vi "tower Check for New Command.vi"(8 "Current Command":T6, 10 "Wait time (ms)":dbl, 11 "Finished?":bool) -> (0 "Completion":T4, 1 "Subsystem Name":string, 2 "Current Command":T1, 3 "Initial Trace String":string, 4 "NextCommand":T6)   [LabVIEW 2017]
doc: "This VI is called for each controller loop iteration. It checks for new commands, updates timing data, and upon completion, notifies any waiting commands."
uses:
  tower Setpoints.ctl
  tower Operations.ctl
  <vilib>/Rock Robotics/WPI/Framework/Command Status Info.ctl
  <vilib>/Rock Robotics/WPI/Framework/Completion Status.ctl
  <vilib>/Rock Robotics/WPI/Framework/Completion Notifier.ctl
  tower Published Globals.vi
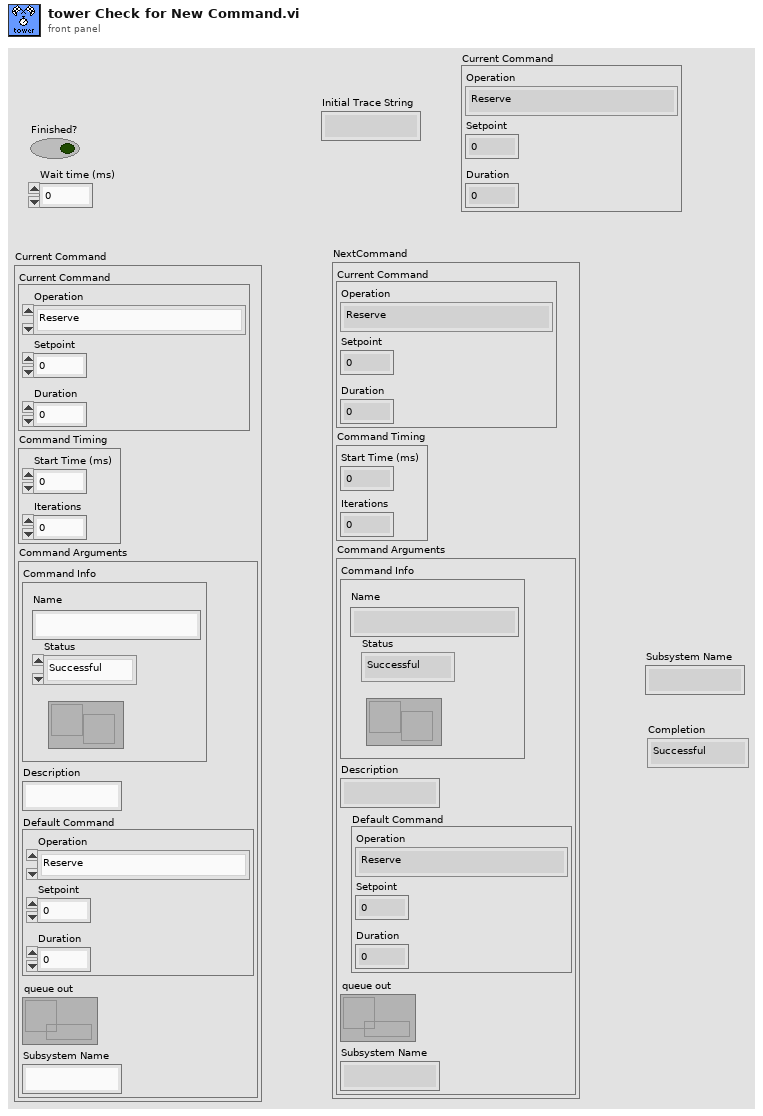
[diagram p1: front panel]
types:
  T1 = typedef "tower Setpoints.ctl" = cluster{"Operation":T2, "Setpoint":dbl, "Duration":dbl}
  T2 = typedef "tower Operations.ctl" = enum16{"Reserve", "Read Current", "Immediate", "LaunchClimber", "ArmReset", "ArmPosition", "TowerClimbImmediate", "ArmSpitPosition", "ClimbArmMove"}
  T3 = typedef "Command Status Info.ctl" = cluster{"Name":string, "Status":T4, "notifier out":T5}
  T4 = typedef "Completion Status.ctl" = enum16{"Successful", "Aborted", "Incomplete"}
  T5 = typedef "Completion Notifier.ctl" = refnum<notifier>
  T6 = cluster{"Current Command":T1, "Command Timing":cluster{"Start Time (ms)":u32, "Iterations":i32}, "Command Arguments":cluster{"Command Info":T3, "Description":string, "Default Command":T1, "queue out":refnum<queue>, "Subsystem Name":string}}
  T7 = cluster{"Command Info":T3, "Description":string, "Default Command":T1, "queue out":refnum<queue>, "Subsystem Name":string}
  T8 = cluster{"Default Command":T1, "Command Info":T3, "Description":string}
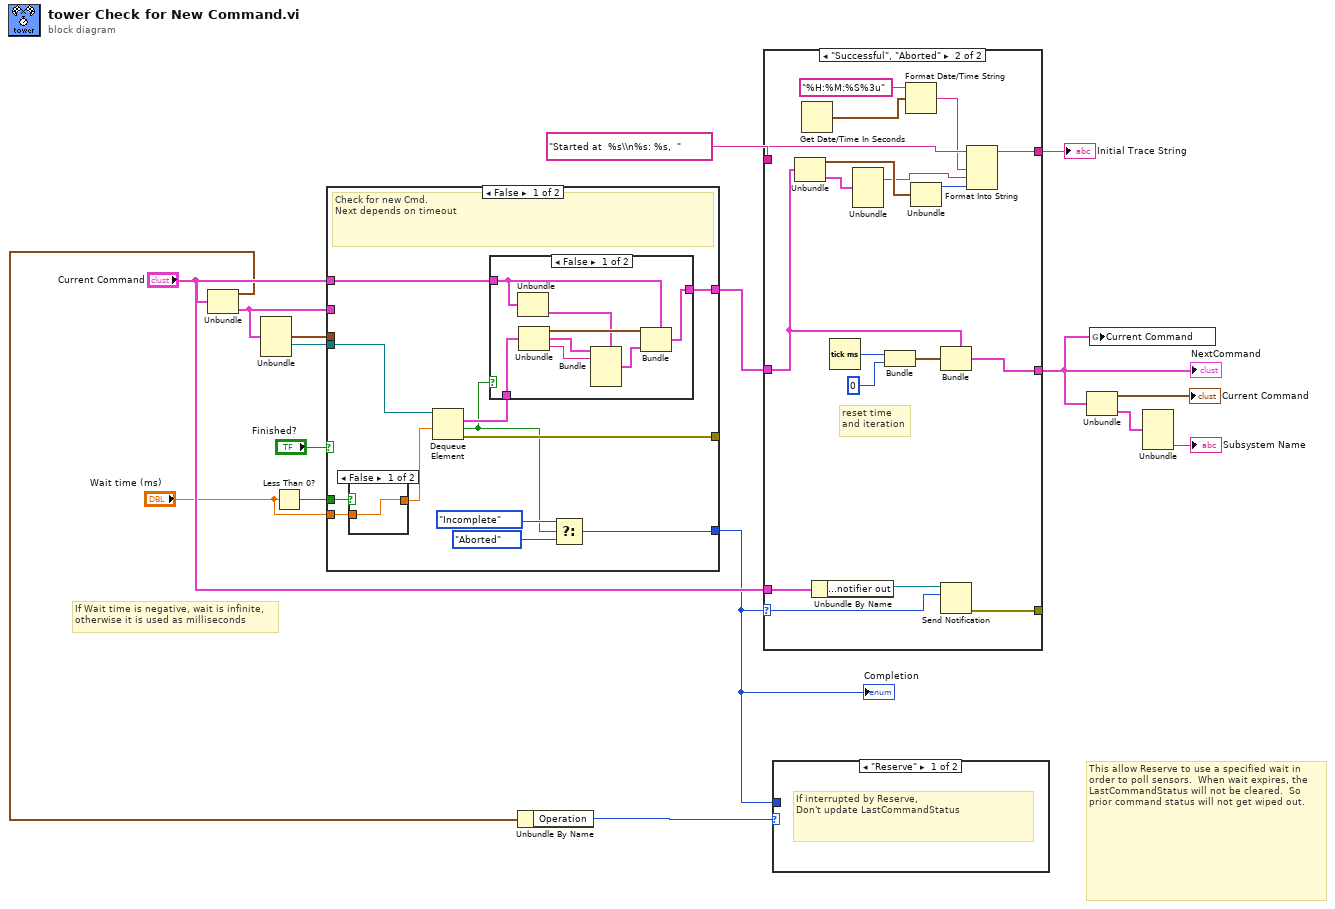
[diagram p0: block diagram]
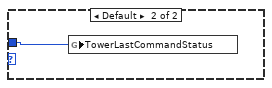
[diagram p2: hidden frame]
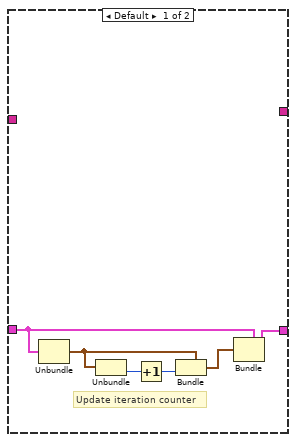
[diagram p3: hidden frame]
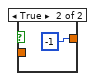
[diagram p5: hidden frame]
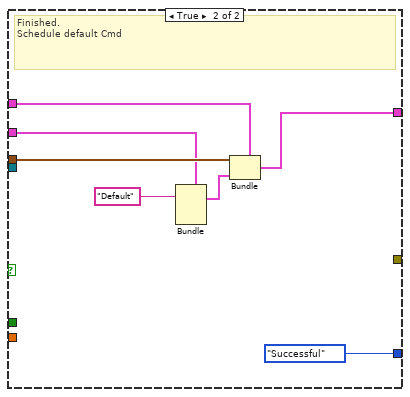
[diagram p6: hidden frame]
diagram:
  # "This allow Reserve to use a specified wait in order to poll sensors.  When wait expires, the LastCommandStatus will not be cleared.  So prior command status will not get wiped out."
  # "If Wait time is negative, wait is infinite,\notherwise it is used as milliseconds"
  n1 = Unbundle("Current Command") -> ("Current Command"=w2:T1, "Command Arguments"=w7:T7)  [unwired: 1 out]
  n2 = Unbundle(w7) -> ("Default Command"=w10:T1, "queue out"=w11:refnum<queue>)  [unwired: 3 out]
  n3 = Less Than 0?(x="Wait time (ms)") -> (x < 0?=w5:bool)
  n4 = case shown="False" "Finished?" {
    tunnel: [w24 w46] -> w14
    tunnel: w5 -> [w26 _]
    tunnel: [w29 Completion_Status."Successful"] -> w3
    tunnel: [w21 _] -> _
    tunnel: w11 -> [w23 _]
    tunnel: "Current Command" -> [w25 w45]
    tunnel: w10 -> [_ w44]
    tunnel: w7 -> [_ w42]
    tunnel: "Wait time (ms)" -> [w18 _]
    frame False {
      # "Check for new Cmd.\nNext depends on timeout"
      n5 = case shown="False" w26 {
        tunnel: [w39 -1] -> w22
        tunnel: w18 -> [w39 _]
        frame False {
        }
        frame True {
        }
      }
      n6 = Dequeue Element(queue=w23, timeout in ms (-1)=w22) -> (element=w20:T8, timed out?=w19:bool, error out=w21:errorcluster)  [unwired: 1 in, 1 out]
      n7 = case shown="False" w19 {
        tunnel: w20 -> [w37 _]
        tunnel: w25 -> [w34 w38]
        tunnel: [w30 w38] -> w24
        frame False {
          n8 = Unbundle(w34) -> ("Command Arguments"=w33:T7)  [unwired: 2 out]
          n9 = Unbundle(w37) -> ("Default Command"=w36:T1, "Command Info"=w31:T3, "Description"=w32:string)
          n10 = Bundle(cluster=w33, "Command Info"=w31, "Description"=w32) -> (w35:T7)  [unwired: 3 in]
          n11 = Bundle(cluster=w34, "Current Command"=w36, "Command Arguments"=w35) -> (w30:T6)  [unwired: 1 in]
        }
        frame True {
        }
      }
      n12 = Select(t=Completion_Status."Incomplete", s=w19, f=Completion_Status."Aborted") -> (s? t:f=w29:T4)
    }
    frame True {
      # "Finished.\nSchedule default Cmd"
      n13 = Bundle(cluster=w42, "Description"="Default") -> (w43:T7)  [unwired: 4 in]
      n14 = Bundle(cluster=w45, "Current Command"=w44, "Command Arguments"=w43) -> (w46:T6)  [unwired: 1 in]
    }
  }
  "Completion" <- w3
  n15 = Unbundle By Name(w2) -> ("Operation"=w1:T2)
  n16 = case shown="\"Successful\", \"Aborted\"" w3 {
    selector: w3 -> [_ w71]
    tunnel: "Current Command" -> [_ w68]
    tunnel: "Started at  %s\\n%s: %s,  " ("format string") -> [_ w67]
    tunnel: [_ w66] -> w16
    tunnel: w14 -> [w50 w55]
    tunnel: [w51 w62] -> w6
    tunnel: [_ w59] -> _
    frame Default {
      # "Update iteration counter"
      n17 = Unbundle(w50) -> ("Command Timing"=w49:cluster{"Start Time (ms)":u32, "Iterations":i32})  [unwired: 2 out]
      n18 = Unbundle(w49) -> ("Iterations"=w52:i32)  [unwired: 1 out]
      n19 = Increment(x=w52) -> (x+1=w53:i32)
      n20 = Bundle(cluster=w49, "Iterations"=w53) -> (w48:cluster{"Start Time (ms)":u32, "Iterations":i32})  [unwired: 1 in]
      n21 = Bundle(cluster=w50, "Command Timing"=w48) -> (w51:T6)  [unwired: 2 in]
    }
    frame "Successful", "Aborted" {
      # "reset time\nand iteration"
      n22 = Unbundle(w55) -> ("Current Command"=w65:T1, "Command Arguments"=w60:T7)  [unwired: 1 out]
      n23 = Get Date/Time In Seconds() -> (seconds since 1Jan1904=w58:timestamp)
      n24 = Unbundle By Name(w68) -> ("Command Arguments.Command Info.notifier out"=w70:T5)
      n25 = Tick Count (ms)() -> (millisecond timer value=w64:u32)
      n26 = Unbundle(w60) -> ("Description"=w57:string)  [unwired: 4 out]
      n27 = Bundle("millisecond timer value"=w64, 0) -> (w61:cluster{"millisecond timer value":u32, i32})  [unwired: 1 in]
      n28 = Format Date/Time String(time format string (%c)="%H:%M:%S%3u", seconds (now)=w58) -> (date/time string=w56:string)  [unwired: 1 in]
      n29 = Unbundle(w65) -> ("Operation"=w69:T2)  [unwired: 2 out]
      n30 = Bundle(cluster=w55, "Command Timing"=w61) -> (w62:T6)  [unwired: 2 in]
      n31 = Send Notification(notification=w71, notifier=w70) -> (error out=w59:errorcluster)  [unwired: 1 in, 1 out]
      n32 = Format Into String(format string=w67, w56, w57, w69) -> (resulting string=w66:string)  [unwired: 2 in, 1 out]
    }
  }
  "NextCommand" <- w6
  "Initial Trace String" <- w16
  n33 = case shown="\"Reserve\"" w1 {
    tunnel: w3 -> [_ w72]
    frame "Reserve" {
      # "If interrupted by Reserve,\nDon't update LastCommandStatus"
    }
    frame Default {
      n34 = global write "tower Published Globals.vi" "TowerLastCommandStatus"(w72) -> ()
    }
  }
  n35 = Unbundle(w6) -> ("Current Command"=→"Current Command":T1, "Command Arguments"=w9:T7)  [unwired: 1 out]
  n36 = global write "tower Published Globals.vi" "Current Command"(w6) -> ()
  n37 = Unbundle(w9) -> ("Subsystem Name"=→"Subsystem Name":string)  [unwired: 4 out]
